vi "FT_Write_Byte_Data.vi"(2 "Bytes To Write":u32, 3 "Buffer":u8[](array[numeric]), 4 "Handle":u32) -> (0 "Bytes Written":u32, 1 "FT_Status":u32(ring) items=["FT_OK", "FT_INVALID_HANDLE", "FT_DEVICE_NOT_FOUND", "FT_DEVICE_NOT_OPENED", "FT_IO_ERROR", "FT_INSUFFICIENT_RESOURCES", "FT_INVALID_PARAMETER", "FT_INVALID_BAUD_RATE", "FT_DEVICE_NOT_OPENED_FOR_ERASE", "FT_DEVICE_NOT_OPENED_FOR_WRITE", "FT_FAILED_TO_WRITE_DEVICE", "FT_EEPROM_READ_FAILED", "FT_EEPROM_WRITE_FAILED", "FT_EEPROM_ERASE_FAILED", "FT_EEPROM_NOT_PRESENT", "FT_EEPROM_NOT_PROGRAMMED", "FT_INVALID_ARGS", "FT_NOT_SUPPORTED", "FT_OTHER_ERROR"])   [LabVIEW 2011]
uses:
  ftd2xx.dll
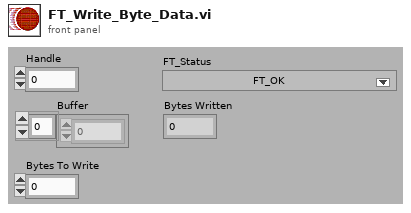
[diagram p1: front panel]
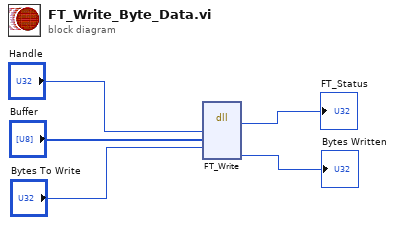
[diagram p0: block diagram]
diagram:
  n1 = dll-call lib="C:/Users/INL Students/Desktop/INL labview repository/3rd Party/D2XX_Functions_7.0/FTD2XX.dll" fn="FT_Write"("Handle"="Handle", "Buffer"="Buffer", "BytesToWrite"="Bytes To Write") -> ("FT_Status"=→"FT_Status":u32, "BytesWritten"=→"Bytes Written":u32)  [unwired: 7 in, 2 out]
